vi "OdczytStanuPowietrza.vi"() -> (0 "Wartoœæ":dbl)   [LabVIEW 2024]
uses:
  <vilib>/httpClient/LabVIEWHTTPClient.lvlib
panel:
  in  "Zapasowy URL":string="https://api.waqi.info/feed/A91057/?token=f76e8feceb7861a021351fe865ea9606d21fcc94"
  out "API w JSON":string
  in  "URL":string="https://api.waqi.info/feed/A91057/?token=cfb339186a93ded7695c0cbf3bf53695fd55efc7"
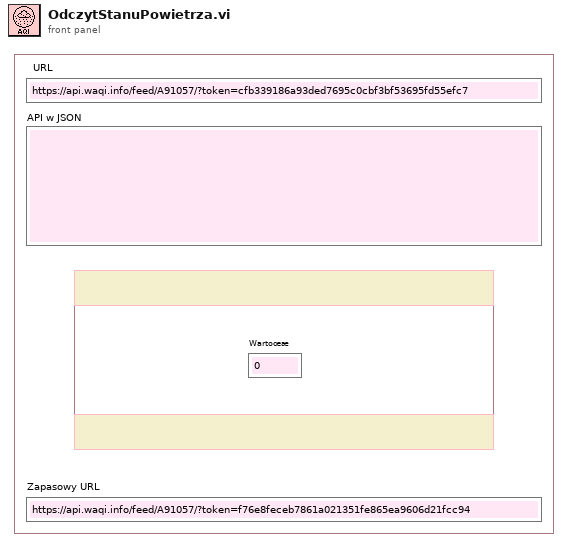
[diagram p1: front panel]
types:
  T1 = typedef "LabVIEWHTTPClient.lvlib/ClientHandle.ctl" = refnum<k1>
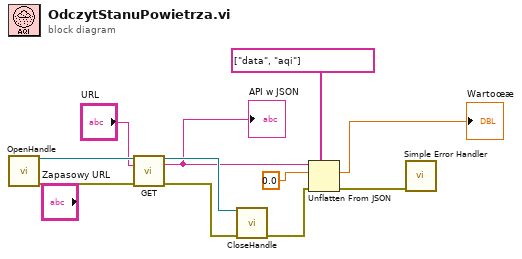
[diagram p0: block diagram]
diagram:
  n1 = call <vilib>:"OpenHandle.vi"() -> ("client handle out"=w11:T1, "error out"=w10:errorcluster)  [unwired: 14 in]
  n2 = call <vilib>:"GET.vi"("client handle"=w11, "url"="URL", "error in (no error)"=w10) -> ("client handle out"=w7:T1, "body"=w3:string, "error out"=w8:errorcluster)  [unwired: 9 in, 1 out]
  "API w JSON" <- w3
  n3 = call <vilib>:"CloseHandle.vi"("client handle"=w7, "error in (no error)"=w8) -> ("error out"=w2:errorcluster)  [unwired: 13 in]
  n4 = Unflatten From JSON(path=string[] ["data", "aqi"], JSON string=w3, type and defaults=0.0, error in (no error)=w2) -> (value=→"Wartoœæ":dbl, error out=w6:errorcluster)  [unwired: 3 in]
  n5 = call <vilib>:"Simple Error Handler.vi"("error in (no error)"=w6) -> ()  [unwired: 4 in, 5 out]
